vi "toggle.vi"(11 "Boolean in":bool) -> (3 "Boolean out":bool)   [LabVIEW 2015]
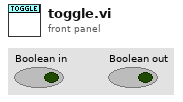
[diagram p1: front panel]
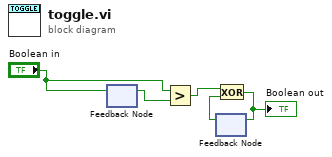
[diagram p0: block diagram]
diagram:
  n1 = feedback #1() -> (w2:bool)  [unwired: 1 in]
  n2 = feedback-in #1("Boolean in") -> ()
  n3 = Greater?(x="Boolean in", y=w2) -> (0:w1:bool)
  n4 = feedback #2() -> (w4:bool)  [unwired: 1 in]
  n5 = Exclusive Or(1:w4, 2:w1) -> (0:w5:bool)
  "Boolean out" <- w5
  n6 = feedback-in #2(w5) -> ()
